vi "zad3.vi"() -> ()   [LabVIEW 2018]
panel:
  in  "Format (44kHz, 16Bit, stereo)":cluster{"Rate":i32, "Bits":i32, "Channels":u32}={"Rate"=48000, "Bits"=16, "Channels"=2}
  in  "Buffer Config":T1={"# buffers"=4, "Buffer size"=600, "unit (ms)"=enum."Samples"}
  out "Waveform Graph":i32[][](graph)
  in  "idev":u32
  in  "?":bool
  in  "Play":bool
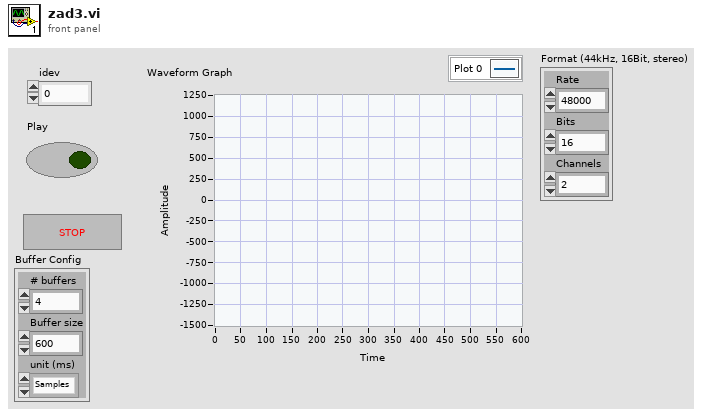
[diagram p1: front panel]
types:
  T1 = cluster{"# buffers":i32, "Buffer size":i32, "unit (ms)":enum16{"time (ms)", "Samples"}}
  T2 = enum16{"Idle", "Initialization", "Acquisition", "End"}
  T3 = typedef "SoundHandle.ctl" = cluster{"DeviceID":u16, "Samples/buf":u32, "Sampl rate":u32, "Bits/sample":u16, "Channels":u8, "Opened":bool}
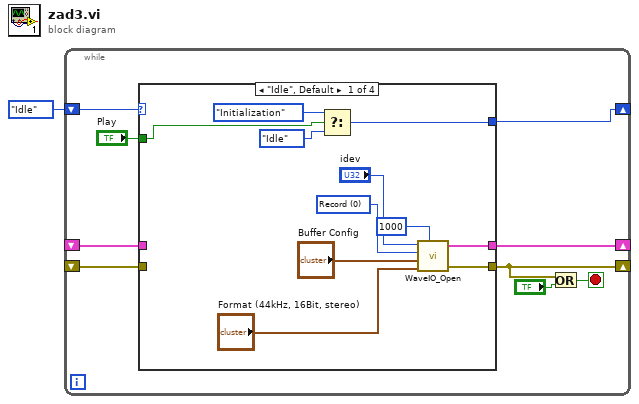
[diagram p0: block diagram]
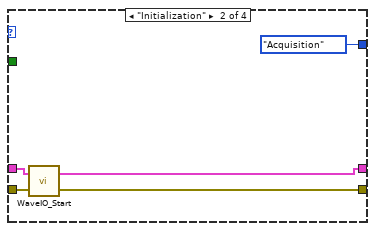
[diagram p2: hidden frame]
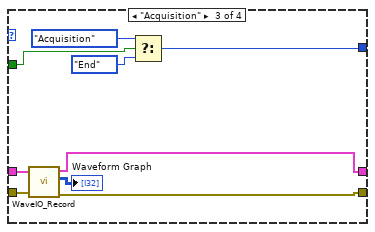
[diagram p3: hidden frame]
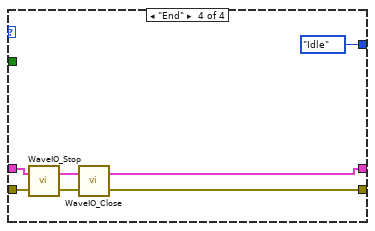
[diagram p4: hidden frame]
diagram:
  n1 = while {
    shift-right: [w8] -> _
    shift-left: T2."Idle" -> [w10]
    shift-right: [w5] -> _
    shift-left: _ -> [w4]
    shift-right: [w2] -> _
    shift-left: _ -> [w3]
    stop <- w7 stop-if-true
    n2 = case shown="\"Idle\", Default" w10 {
      tunnel: "Play" -> [w21 _ w34 _]
      tunnel: [w18 T2."Acquisition" w35 T2."Idle"] -> w8
      tunnel: [w12 w23 w28 w36] -> w5
      tunnel: [w11 w22 w27 w37] -> w2
      tunnel: w4 -> [_ w25 w31 w41]
      tunnel: w3 -> [_ w24 w30 w40]
      frame "Idle", Default {
        w15 = u16 0 items=["Record", "Play", "Loopback", "ASIO input", "ASIO output", "Record (WASAPI)", "Play (WASAPI)", "Record Combi", "Play Combi"] ("device type (Record)")
        n3 = Select(t=T2."Initialization", s=w21, f=T2."Idle") -> (s? t:f=w18:T2)
        n4 = call "WaveIO_Open.vi"("idev"="idev", "Watchdog timeout (msec) (default=OFF)"=u32 1000 ("milliseconds to wait"), "device type (Record)"=w15, "Buffer Config"="Buffer Config", "Format (44kHz, 16Bit, stereo)"="Format (44kHz, 16Bit, stereo)") -> ("Sound Handle Out"=w12:T3, "error out"=w11:errorcluster)  [unwired: 2 in]
      }
      frame "Initialization" {
        n5 = call "WaveIO_Start.vi"("error in (no error)"=w24, "Handle"=w25) -> ("error out"=w22:errorcluster, "Handle Out"=w23:T3)
      }
      frame "Acquisition" {
        n6 = call "WaveIO_Record.vi"("Handle"=w31, "error in (no error)"=w30) -> ("Handle Out"=w28:T3, "Data"=→"Waveform Graph":i32[][], "error out"=w27:errorcluster)  [unwired: 1 in, 2 out]
        n7 = Select(t=T2."Acquisition", s=w34, f=T2."End") -> (s? t:f=w35:T2)
      }
      frame "End" {
        n8 = call "WaveIO_Stop.vi"("error in (no error)"=w40, "Handle"=w41) -> ("error out"=w38:errorcluster, "Handle Out"=w39:T3)
        n9 = call "WaveIO_Close.vi"("error in (no error)"=w38, "Handle"=w39) -> ("error out"=w37:errorcluster, "Handle Out"=w36:T3)
      }
    }
    n10 = Or(x=w2, y="?") -> (x .or. y?=w7:bool)
  }
